vi "Path Planner 3.vi"(11 "GIC Input":T1={"Real/Sim"=FALSE, "WP Lats and Longs"={"WP Lats"=[], "WP Longs"=[]}, "GPS Time Int"=0.0, "GPS Com Port"="", "Compass Com Port"="", "Prop Com Port"="", "GPS Data"=[], "Compass"=0.0, "LMS Vector"=[], "Vision Vector"=[], "Direction Cmd"=0.0, "Speed Cmd"=0.0, "Time of Last GPS"=0.0, "WP Vector"=[], "WP Number"=0, "Num of WPs"=0, "SW Map"=[], "Obst Lats and Longs"={"Obst Lats"=[], "Obst Longs"=[]}, "Parameters"=[], "Path Cluster"={"Path x nodes"=[], "Path y nodes"=[]}, "     Use ?\nOff       On"=[TRUE, TRUE, FALSE, FALSE]} {"Obst Lats and Longs"."Obst Longs" format="%#_8g"; "Obst Lats and Longs"."Obst Lats" format="%#_8g"}) -> (3 "GIC Output":T1={"Real/Sim"=FALSE, "WP Lats and Longs"={"WP Lats"=[], "WP Longs"=[]}, "GPS Time Int"=0.0, "GPS Com Port"="", "Compass Com Port"="", "Prop Com Port"="", "GPS Data"=[], "Compass"=0.0, "LMS Vector"=[], "Vision Vector"=[], "Direction Cmd"=0.0, "Speed Cmd"=0.0, "Time of Last GPS"=0.0, "WP Vector"=[], "WP Number"=0, "Num of WPs"=0, "SW Map"=[], "Obst Lats and Longs"={"Obst Lats"=[], "Obst Longs"=[]}, "Parameters"=[], "Path Cluster"={"Path x nodes"=[], "Path y nodes"=[]}, "     Use ?\nOff       On"=[TRUE, TRUE, FALSE, FALSE]} {"Obst Lats and Longs"."Obst Longs" format="%#_8g"; "Obst Lats and Longs"."Obst Lats" format="%#_8g"})   [LabVIEW 2014]
panel:
  out "goaly rip":dbl
  out "goalx rip":dbl
  out "SWMap":dbl[][](array[numeric])
  out "goal y":dbl=1.0
  out "goal x":dbl=1.0
  # "GPS"
  # "LMS"
  # "Vision"
  # "Prop"
  # "GPS"
  # "LMS"
  # "Vision"
  # "Prop"
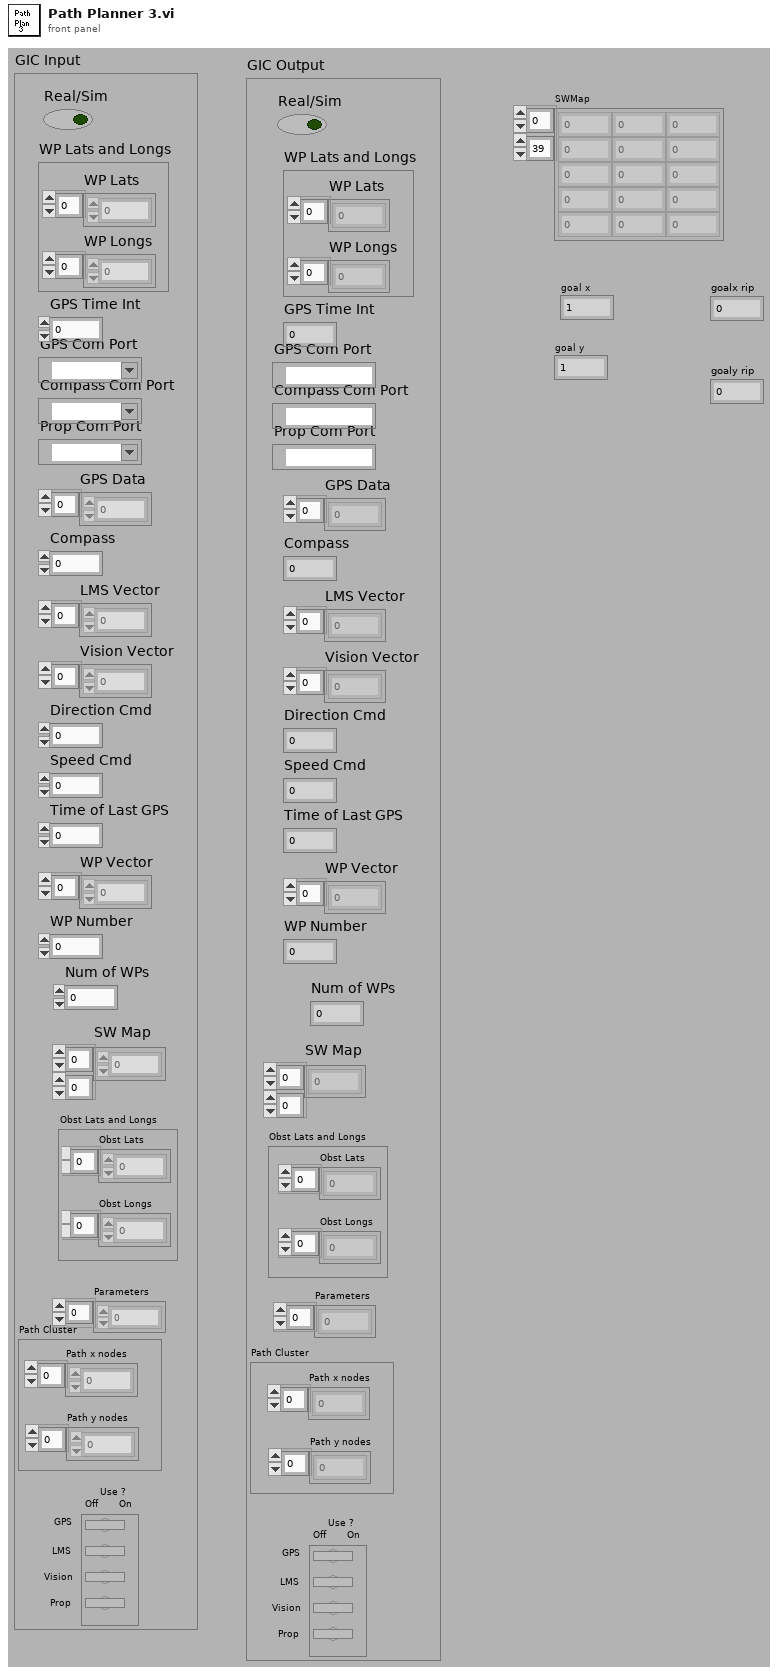
[diagram p1: front panel]
types:
  T1 = cluster{"Real/Sim":bool, "WP Lats and Longs":cluster{"WP Lats":dbl[], "WP Longs":dbl[]}, "GPS Time Int":dbl, "GPS Com Port":refnum<visa-resource-name>, "Compass Com Port":refnum<visa-resource-name>, "Prop Com Port":refnum<visa-resource-name>, "GPS Data":dbl[], "Compass":dbl, "LMS Vector":dbl[], "Vision Vector":dbl[], "Direction Cmd":dbl, "Speed Cmd":dbl, "Time of Last GPS":dbl, "WP Vector":dbl[], "WP Number":i32, "Num of WPs":i16, "SW Map":i32[][], "Obst Lats and Longs":cluster{"Obst Lats":dbl[], "Obst Longs":dbl[]}, "Parameters":dbl[], "Path Cluster":cluster{"Path x nodes":dbl[], "Path y nodes":dbl[]}, "     Use ?\nOff       On":bool[]}
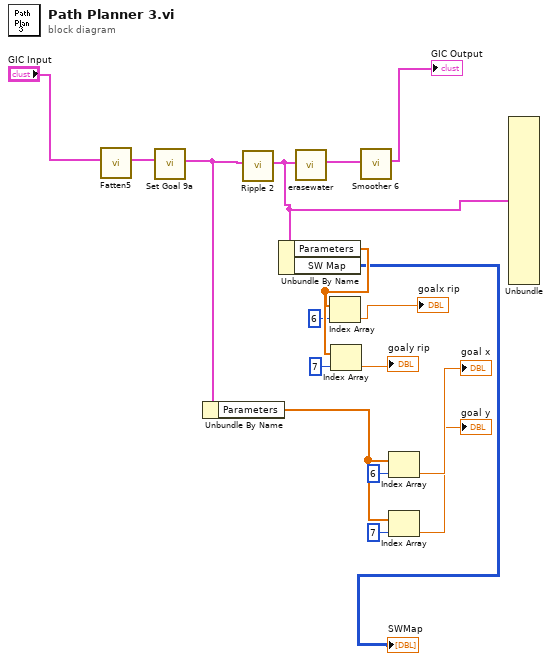
[diagram p0: block diagram]
diagram:
  n1 = call "Fatten5.vi"("GIC Input"="GIC Input") -> ("GIC Output"=w9:T1)  [unwired: 10 in]
  n2 = call "Set Goal 9a.vi"("GIC Input"=w9) -> ("GIC Output"=w8:T1)  [unwired: 10 in]
  n3 = Unbundle By Name(w8) -> ("Parameters"=w16:dbl[])
  n4 = call "Ripple 2.vi"("GIC Input"=w8) -> ("GIC Output"=w7:T1)  [unwired: 10 in]
  n5 = Unbundle By Name(w7) -> ("Parameters"=w6:dbl[], "SW Map"=→"SWMap":i32[][])
  n6 = call "erasewater.vi"("GIC Input"=w7) -> ("GIC Output"=w11:T1)  [unwired: 10 in]
  n7 = Index Array(array=w6, index=6) -> (element=→"goalx rip":dbl)
  n8 = Index Array(array=w6, index=7) -> (element=→"goaly rip":dbl)
  n9 = call "Smoother 6.vi"("GIC Input"=w11) -> ("GIC Output"=→"GIC Output":T1)  [unwired: 10 in]
  n10 = Index Array(array=w16, index=6) -> (element=→"goal x":dbl)
  n11 = Index Array(array=w16, index=7) -> (element=→"goal y":dbl)
  n12 = Unbundle(w7) -> ()  [unwired: 21 out]
